vi "Radio Label Tester.vi"(10 "Radio Labels":i32[](array[numeric]), 11 "Graph Matrix":T1) -> (3 "Works?":bool)   [LabVIEW 2016]
uses:
  <vilib>/Analysis/Matrix/Datatypes/RealMatrix.ctl
  <vilib>/Analysis/Matrix/NI_Matrix.lvlib
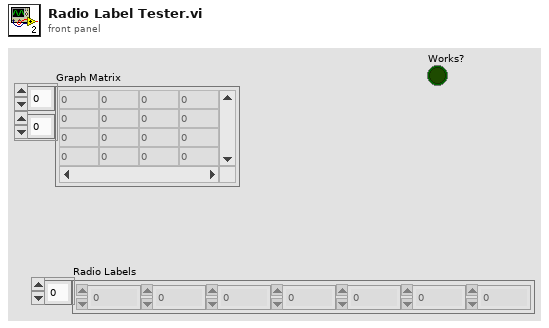
[diagram p1: front panel]
types:
  T1 = typedef "NI_Matrix.lvlib/RealMatrix.ctl" = dbl[][]
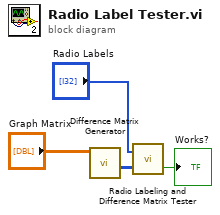
[diagram p0: block diagram]
diagram:
  n1 = call "Difference Matrix Generator.vi"("Graph Matrix"="Graph Matrix") -> ("Difference Between Labels Matrix"=w3:i32[][])  [unwired: 7 in, 3 out]
  n2 = call "Radio Labeling and Difference Matrix Tester.vi"("Difference Between Labels Matrix"=w3, "Radio Labels"="Radio Labels") -> ("Works?"=→"Works?":bool)  [unwired: 1 out]
